vi "PreCalc Frame Durations.vi"(8 "error in (no error)":errorcluster, 9 "FD Baud Rate":u64=1000000, 10 "Baud Rate":u64=125000, 11 "CAN Bus Class In":refnum<class "CANBus_Load_Calculator.lvclass">) -> (0 "error out":errorcluster, 3 "CAN Bus Class Out":refnum<class "CANBus_Load_Calculator.lvclass">)   [LabVIEW 2018, in "NI-XNET Monitor Engine.lvlib" / "XNET-Bus-Load-Calculator.lvlib" / "CANBus_Load_Calculator.lvclass"]
uses:
  CANBus_Load_Calculator.lvclass
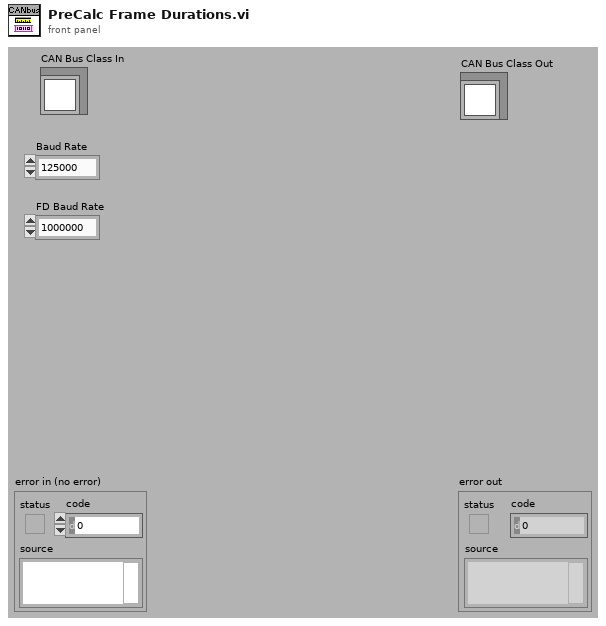
[diagram p1: front panel]
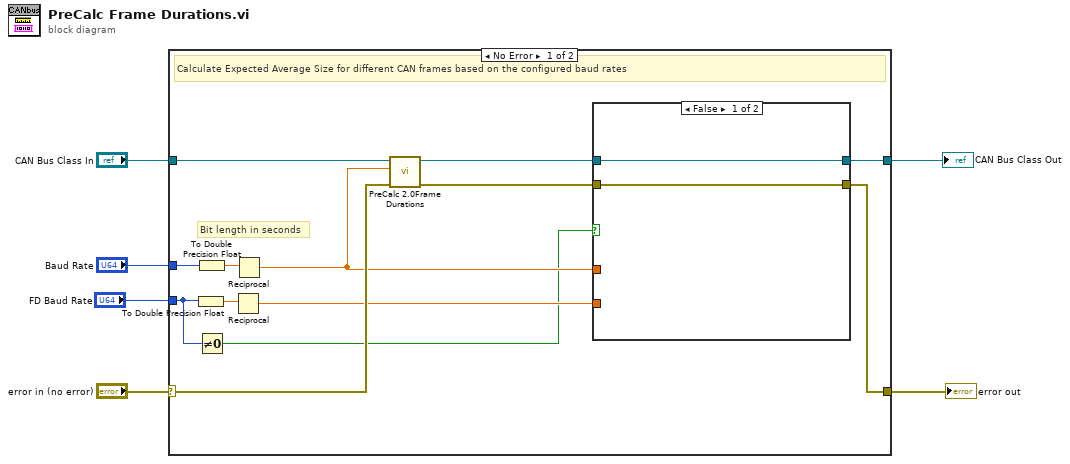
[diagram p0: block diagram]
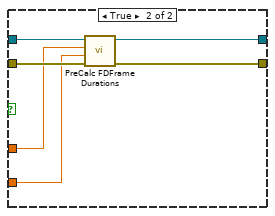
[diagram p2: hidden frame]
diagram:
  n1 = case shown="No Error" "error in (no error)" {
    selector: "error in (no error)" -> [w16 w29]
    tunnel: [w12 w29] -> w5
    tunnel: "Baud Rate" -> [w19 _]
    tunnel: "CAN Bus Class In" -> [w17 w28]
    tunnel: [w14 w28] -> w2
    tunnel: "FD Baud Rate" -> [w8 _]
    frame No Error {
      # "Bit length in seconds"
      # "Calculate Expected Average Size for different CAN frames based on the configured baud rates"
      n2 = To Double Precision Float(number=w8) -> (double precision float=w9:dbl)
      n3 = To Double Precision Float(number=w19) -> (double precision float=w18:dbl)
      n4 = Not Equal To 0?(x=w8) -> (x != 0?=w7:bool)
      n5 = Reciprocal(x=w9) -> (1/x=w10:dbl)
      n6 = Reciprocal(x=w18) -> (1/x=w11:dbl)
      n7 = call "PreCalc 2.0Frame Durations.vi"("error in (no error)"=w16, "Bit Time (seconds)"=w11, "CANBus_Load_Calculator in"=w17) -> ("error out"=w13:errorcluster, "CANBus_Load_Calculator out"=w15:refnum<class "CANBus_Load_Calculator.lvclass">)  [unwired: 7 in]
      n8 = case shown="False" w7 {
        tunnel: w15 -> [w21 w27]
        tunnel: [w21 w26] -> w14
        tunnel: w13 -> [w20 w25]
        tunnel: [w20 w24] -> w12
        tunnel: w11 -> [_ w23]
        tunnel: w10 -> [_ w22]
        frame False {
        }
        frame True {
          n9 = call "PreCalc FDFrame Durations.vi"("error in (no error)"=w25, "Bit Time FD (seconds)"=w22, "Bit Time (seconds)"=w23, "CANBus_Load_Calculator in"=w27) -> ("error out"=w24:errorcluster, "CANBus_Load_Calculator out"=w26:refnum<class "CANBus_Load_Calculator.lvclass">)  [unwired: 6 in]
        }
      }
    }
    frame Error {
    }
  }
  "CAN Bus Class Out" <- w2
  "error out" <- w5
